vi "Read Background Image.vi"(9 "Pane in":refnum<class "Pane.lvclass">) -> (3 "Pane out":refnum<class "Pane.lvclass">, 4 "image data":T1)   [LabVIEW 2014, in "Pane.lvclass"]
uses:
  Pane.lvclass
  <vilib>/picture/picture.llb/imagedata.ctl
  Pane.lvclass/Pane.ctl
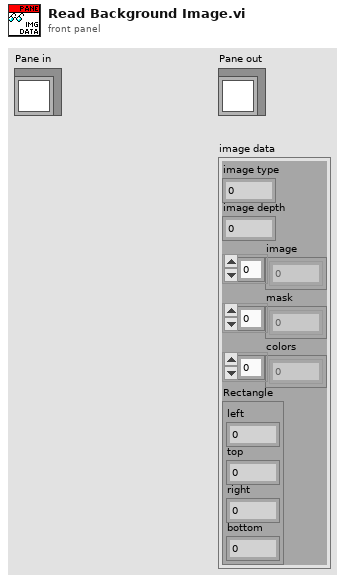
[diagram p1: front panel]
types:
  T1 = typedef "imagedata.ctl" = cluster{"image type":i32, "image depth":i32, "image":u8[], "mask":u8[], "colors":u32[], "Rectangle":cluster{"left":i16, "top":i16, "right":i16, "bottom":i16}}
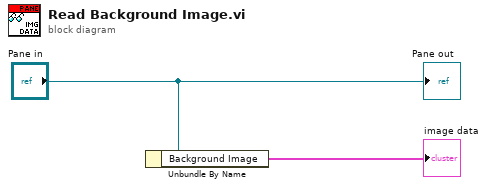
[diagram p0: block diagram]
diagram:
  n1 = Unbundle By Name("Pane in") -> ("Background Image"=→"image data":T1)
  "Pane out" <- "Pane in"
